vi "SVXMPL_Set Panel Size.vi"(6 "Front Panel Window:Window Bounds":T1={"left"=0, "top"=0, "right"=800, "bottom"=600}) -> (4 "error out":errorcluster)   [LabVIEW 2017]
panel:
  out "Top Level Caller":string
  in  "error in (no error)":errorcluster
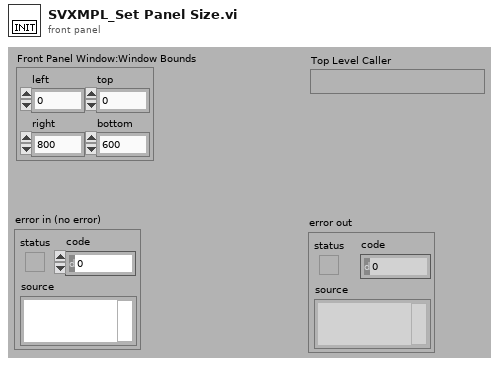
[diagram p1: front panel]
types:
  T1 = cluster{"left":i16, "top":i16, "right":i16, "bottom":i16}
  T2 = enum32{"invalid app kind", "Development System", "Run Time System", "Student Edition", "Embedded LabVIEW", "Evaluation", "Custom"}
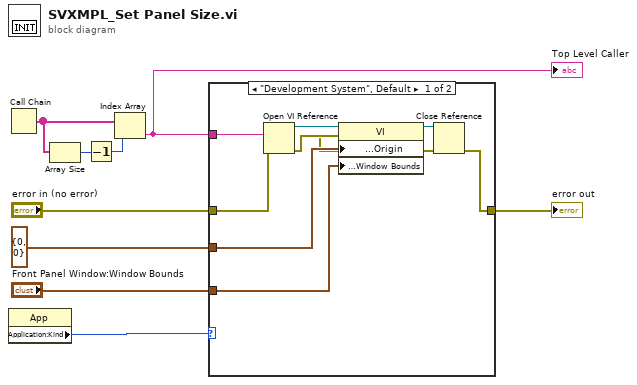
[diagram p0: block diagram]
diagram:
  n1 = Call Chain() -> (call chain=w8:string[])
  n2 = property class="App"() -> ("Application:Kind"=w1:T2)  [unwired: 2 in, 2 out]
  n3 = Array Size(array=w8) -> (size(s)=w9:i32)
  n4 = Decrement(x=w9) -> (x-1=w7:i32)
  n5 = Index Array(array=w8, index=w7) -> (element=w4:string)
  "Top Level Caller" <- w4
  n6 = case shown="\"Development System\", Default" w1 {
    tunnel: "Front Panel Window:Window Bounds" -> [w18 _]
    tunnel: cluster{"Horizontal":i16, "Vertical":i16} {"Horizontal"=0, "Vertical"=0} ("Front Panel Window:Origin") -> [w17 _]
    tunnel: w4 -> [w10 _]
    tunnel: "error in (no error)" -> [w12 w19]
    tunnel: [w11 w19] -> w2
    frame "Development System", Default {
      n7 = Open VI Reference(vi path=w10, error in (no error)=w12) -> (vi reference=w16:refnum<vi>, error out=w15:errorcluster)  [unwired: 4 in]
      n8 = property class="VI"(reference=w16, error in=w15, "Front Panel Window:Origin"=w17, "Front Panel Window:Window Bounds"=w18) -> (reference out=w13:refnum<vi>, error out=w14:errorcluster)
      n9 = Close Reference(reference=w13, error in (no error)=w14) -> (error out=w11:errorcluster)
    }
    frame "Embedded LabVIEW" {
    }
  }
  "error out" <- w2
